vi "WriteToFile.vi"(8 "error in (no error)":errorcluster, 9 "Export string":string, 11 "CGrapherDGML in":refnum<class "CGrapherDGML.lvclass">) -> (0 "error out":errorcluster, 3 "CGrapherDGML out":refnum<class "CGrapherDGML.lvclass">)   [LabVIEW 2020, in "DefaultExtensions.lvlib" / "CGrapherDGML.lvclass"]
uses:
  CGrapherDGML.lvclass
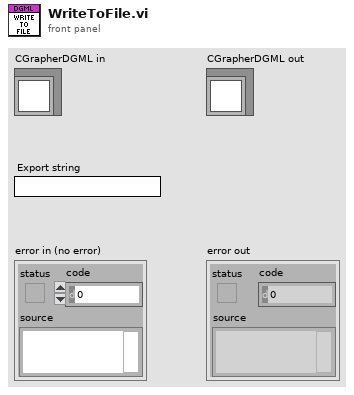
[diagram p1: front panel]
types:
  T1 = enum16{"open", "replace", "create", "open or create", "replace or create", "replace or create with confirmation"}
  T2 = typedef "ExtensionInterfaces.lvlibp/IExporter.lvclass/ExportType.ctl" = enum16{"Dependencies", "Rules", "Invalid dependencies", "Concessions", "Undeclared"}
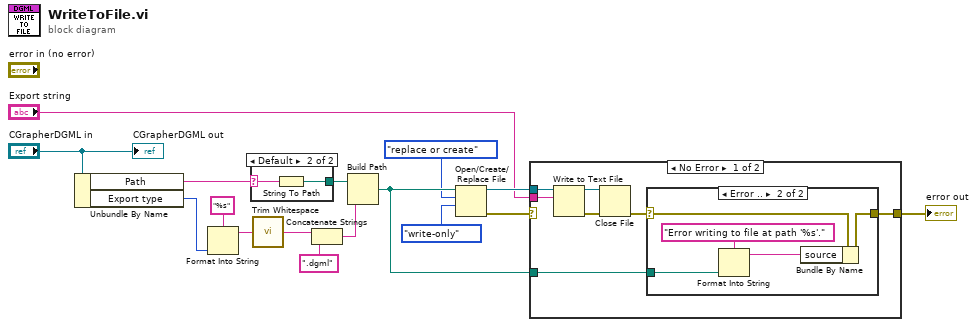
[diagram p0: block diagram]
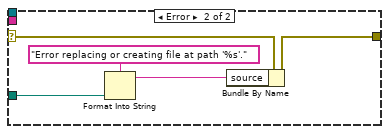
[diagram p3: hidden frame]
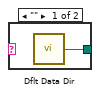
[diagram p4: hidden frame]
diagram:
  n1 = Unbundle By Name("CGrapherDGML in") -> ("Path"=w11:string, "Export type"=w13:T2)
  n2 = Format Into String(format string="%s", w13) -> (resulting string=w14:string)  [unwired: 2 in, 1 out]
  n3 = case shown="Default" w11 {
    selector: w11 -> [_ w18]
    tunnel: [w17 w19] -> w3
    frame "" {
      n4 = call <vilib>:"Dflt Data Dir.vi"() -> ("App:Default Data Directory"=w17:path)
    }
    frame Default {
      n5 = String To Path(string=w18) -> (path=w19:path)
    }
  }
  n6 = call <vilib>:"Trim Whitespace.vi"("string"=w14) -> ("trimmed string"=w12:string)  [unwired: 1 in]
  n7 = Concatenate Strings(w12, ".dgml" ("string")) -> (w2:string)
  n8 = Build Path(base path=w3, name or relative path=w2) -> (appended path=w9:path)
  n9 = Open/Create/Replace File(file path (use dialog)=w9, operation (0:open)=T1."replace or create", access (0:read/write)=enum16{"read/write", "read-only", "write-only"}."write-only") -> (refnum out=w6:refnum<file>, error out=w5:errorcluster)  [unwired: 3 in, 1 out]
  n10 = case shown="No Error" w5 {
    selector: w5 -> [_ w37]
    tunnel: w6 -> [w26 _]
    tunnel: "Export string" -> [w24 _]
    tunnel: [w21 w36] -> w10
    tunnel: w9 -> [w20 w35]
    frame No Error {
      n11 = Write to Text File(file (use dialog)=w26, text=w24) -> (refnum out=w25:refnum<file>, error out=w23:errorcluster)  [unwired: 2 in, 1 out]
      n12 = Close File(refnum=w25, error in=w23) -> (error out=w22:errorcluster)  [unwired: 1 out]
      n13 = case shown="Error .." w22 {
        selector: w22 -> [w27 w30]
        tunnel: [w27 w29] -> w21
        tunnel: w20 -> [_ w28]
        frame No Error {
        }
        frame Error {
          n14 = Format Into String(format string="Error writing to file at path '%s'.", w28) -> (resulting string=w32:string)  [unwired: 2 in, 1 out]
          n15 = Bundle By Name(cluster=w30, "source"=w32) -> (w29:errorcluster)
        }
      }
    }
    frame Error {
      n16 = Format Into String(format string="Error replacing or creating file at path '%s'.", w35) -> (resulting string=w34:string)  [unwired: 2 in, 1 out]
      n17 = Bundle By Name(cluster=w37, "source"=w34) -> (w36:errorcluster)
    }
  }
  "error out" <- w10
  "CGrapherDGML out" <- "CGrapherDGML in"
